vi "meta_writeAllColumnInfo.vi"(8 "error in (no error)":errorcluster, 9 "start row":i32, 10 "Column":T4, 11 "meta file in":T1) -> (0 "error out":errorcluster, 3 "meta file out":T1)   [LabVIEW 2020, in "NI_ExcelFile.lvlib"]
uses:
  <vilib>/express/express shared/NI_ExcelFile/NI_ExcelFile.lvlib
  <vilib>/express/express shared/NI_ExcelFile/Ctrls/meta_file.ctl
  <vilib>/express/express shared/NI_ExcelFile/Ctrls/meta_Block.ctl
  <vilib>/express/express shared/NI_ExcelFile/Ctrls/meta_BlockType.ctl
  <vilib>/express/express shared/NI_ExcelFile/Ctrls/Columns.ctl
  <vilib>/express/express shared/NI_ExcelFile/Ctrls/ColumnInfo.ctl
  <vilib>/express/express shared/NI_ExcelFile/Ctrls/DataType.ctl
  <vilib>/express/express shared/NI_ExcelFile/Ctrls/meta_ColumnInfo.ctl
  <vilib>/express/express shared/NI_ExcelFile/Ctrls/meta_ColumnInfo_2013.ctl
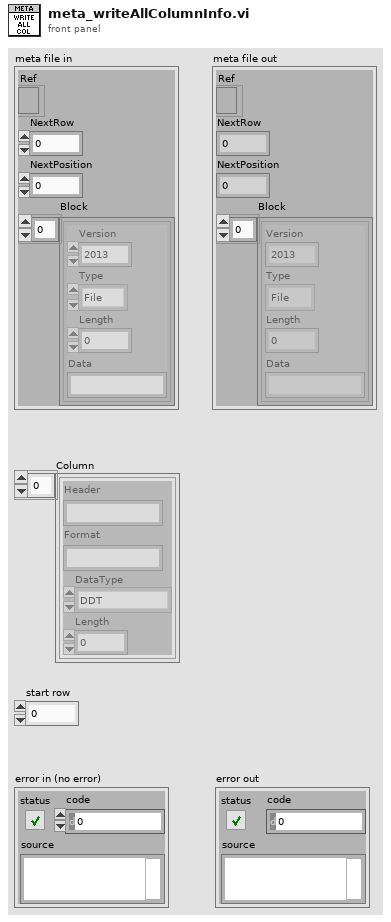
[diagram p1: front panel]
types:
  T1 = typedef "NI_ExcelFile.lvlib/meta_file.ctl" = cluster{"Ref":refnum<file>, "NextRow":i32, "NextPosition":i64, "Block":T2[]}
  T2 = typedef "NI_ExcelFile.lvlib/meta_Block.ctl" = cluster{"Version":u16, "Type":T3, "Length":i32, "Data":string}
  T3 = typedef "NI_ExcelFile.lvlib/meta_BlockType.ctl" = enum16{"NITag", "File", "Column"}
  T4 = typedef "NI_ExcelFile.lvlib/Columns.ctl" = T5[]
  T5 = typedef "NI_ExcelFile.lvlib/ColumnInfo.ctl" = cluster{"Header":string, "Format":string, "DataType":T6, "Length":u64}
  T6 = typedef "NI_ExcelFile.lvlib/DataType.ctl" = enum16{"DDT", "WFM", "Array of STR", "Array of DBL", "Array of I8", "Array of I16", "Array of I32", "Array of I64", "Array of SGL", "Array of U8", "Array of U16", "Array of U32", "Array of U64", "Array of Time"}
  T7 = typedef "NI_ExcelFile.lvlib/meta_ColumnInfo_2013.ctl" = cluster{"Index":i32, "DataType":T6, "Header":string, "Format":string, "StartRow":i32, "Length":i32}
  T8 = typedef "NI_ExcelFile.lvlib/meta_ColumnInfo.ctl" = cluster{"meta_ColumnInfo_2013":T7}
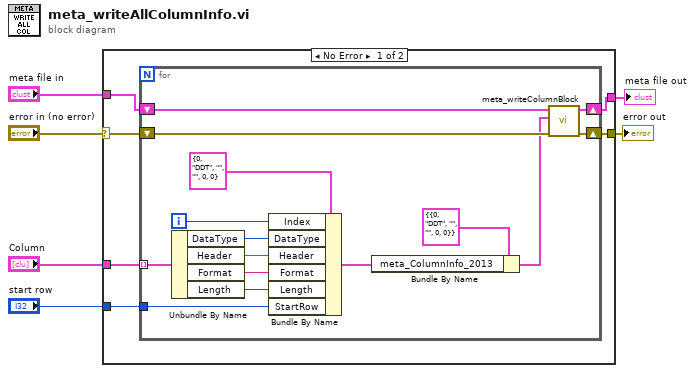
[diagram p0: block diagram]
diagram:
  n1 = case shown="No Error" "error in (no error)" {
    selector: "error in (no error)" -> [w7 w29]
    tunnel: "start row" -> [w12 _]
    tunnel: [w11 w29] -> w5
    tunnel: [w10 w28] -> w4
    tunnel: "Column" -> [w9 _]
    tunnel: "meta file in" -> [w8 w28]
    frame No Error {
      n2 = for {
        shift-right: [w26] -> w11
        shift-left: w7 -> [w27]
        shift-right: [w25] -> w10
        shift-left: w8 -> [w13]
        tunnel: w9 -> [w19] mode=indexing
        tunnel: w12 -> [w14]
        i -> [w20]
        n3 = Unbundle By Name(w19) -> ("DataType"=w16:T6, "Header"=w18:string, "Format"=w17:string, "Length"=w15:u64)
        n4 = Bundle By Name(cluster=T7 {"Index"=0, "DataType"=enum."DDT", "Header"="", "Format"="", "StartRow"=0, "Length"=0} ("meta_ColumnInfo_2013"), "Index"=w20, "DataType"=w16, "Header"=w18, "Format"=w17, "Length"=w15, "StartRow"=w14) -> (w21:T7)
        n5 = Bundle By Name(cluster=T8 {"meta_ColumnInfo_2013"={"Index"=0, "DataType"=enum."DDT", "Header"="", "Format"="", "StartRow"=0, "Length"=0}} ("meta_ColumnInfo"), "meta_ColumnInfo_2013"=w21) -> (w23:T8)
        n6 = call <vilib>:"meta_writeColumnBlock.vi"("error in (no error)"=w27, "meta_ColumnInfo"=w23, "meta file in"=w13) -> ("error out"=w26:errorcluster, "meta file out"=w25:T1)  [unwired: 7 in]
      }
    }
    frame Error {
    }
  }
  "error out" <- w5
  "meta file out" <- w4
